vi "Start TALOS.vi"   [LabVIEW 2020]
uses:
  Circus Launcher TypDef.ctl
panel:
  # "Ladies and Gentlemen,\nplease come in!"
types:
  T1 = typedef "Circus Launcher TypDef.ctl" = refnum<vi>
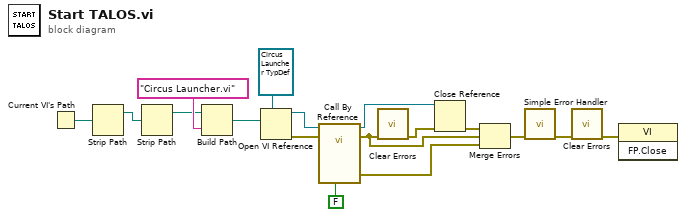
[diagram p0: block diagram]
diagram:
  n1 = Current VI's Path() -> (path=w7:path)
  n2 = Strip Path(path=w7) -> (stripped path=w4:path)  [unwired: 1 out]
  n3 = Strip Path(path=w4) -> (stripped path=w3:path)  [unwired: 1 out]
  n4 = Build Path(base path=w3, name or relative path="Circus Launcher.vi") -> (appended path=w17:path)
  n5 = Open VI Reference(type specifier VI Refnum (for type only)=T1 refnum, vi path=w17) -> (vi reference=w16:T1, error out=w14:errorcluster)  [unwired: 4 in]
  n6 = call-by-ref "?"(reference=w16, error in=w14, "Launch Local?"=FALSE) -> (reference out=w12:T1, error out=w8:errorcluster, 0:"error out"=w13:errorcluster)  [unwired: 10 in]
  n7 = call <vilib>:"Clear Errors.vi"("error in (no error)"=w8) -> ("error out"=w9:errorcluster)  [unwired: 5 in, 1 out]
  n8 = Close Reference(reference=w12, error in (no error)=w9) -> (error out=w11:errorcluster)
  n9 = Merge Errors(w11, w8, w13) -> (w5:errorcluster)
  n10 = call <vilib>:"Simple Error Handler.vi"("error in (no error)"=w5) -> ("error out"=w2:errorcluster)  [unwired: 4 in, 4 out]
  n11 = call <vilib>:"Clear Errors.vi"("error in (no error)"=w2) -> ("error out"=w1:errorcluster)  [unwired: 5 in, 1 out]
  n12 = invoke class="VI" method="FP.Close"(error in=w1) -> ()  [unwired: 2 in, 3 out]
